vi "Send to home.vi"(8 "error in (no error)":errorcluster, 11 "VISA Refnum in":refnum<visa-resource-name>) -> (0 "error out":errorcluster)   [LabVIEW 2020, in "Arduino stepper.lvlib"]
uses:
  Arduino stepper.lvlib
  <vilib>/Instr/_visa.llb/VISA Flush IO Buffer Mask.ctl
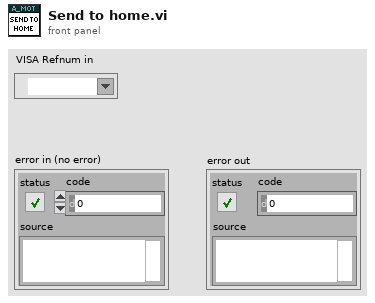
[diagram p1: front panel]
types:
  T1 = typedef "VISA Flush IO Buffer Mask.ctl" = u16
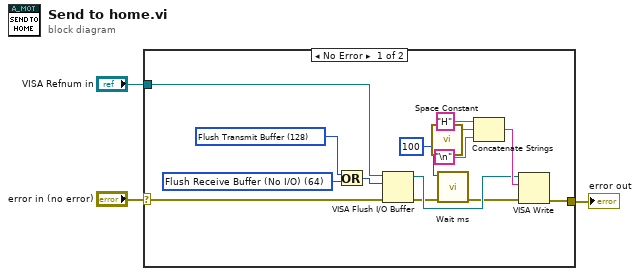
[diagram p0: block diagram]
diagram:
  n1 = case shown="No Error" "error in (no error)" {
    selector: "error in (no error)" -> [w9 w18]
    tunnel: [w4 w18] -> w3
    tunnel: "VISA Refnum in" -> [w11 _]
    frame No Error {
      w6 = T1 64 items=["Flush Receive Buffer"=16, "Write Transmit Buffer to Device"=32, "Flush Receive Buffer (No I/O)"=64, "Flush Transmit Buffer"=128] ("Mask")
      w5 = T1 128 items=["Flush Receive Buffer"=16, "Write Transmit Buffer to Device"=32, "Flush Receive Buffer (No I/O)"=64, "Flush Transmit Buffer"=128] ("Mask")
      n2 = Or(x=w5, y=w6) -> (x .or. y?=w7:T1)
      n3 = VISA Flush I/O Buffer(VISA resource name=w11, mask (16)=w7, error in (no error)=w9) -> (VISA resource name out=w16:refnum<visa-resource-name>, error out=w10:errorcluster)
      n4 = call <vilib>:"Space Constant.vi"() -> ("String"=w8:string)
      n5 = call "Wait ms.vi"("error in (no error)"=w10, "milliseconds to wait"=u32 100) -> ("error out"=w15:errorcluster)  [unwired: 9 in]
      n6 = Concatenate Strings("H" ("string"), w8, "\n") -> (w17:string)
      n7 = VISA Write(VISA resource name=w16, write buffer=w17, error in (no error)=w15) -> (error out=w4:errorcluster)  [unwired: 2 out]
    }
    frame Error {
    }
  }
  "error out" <- w3
